vi "RunJS.vi"() -> ()   [LabVIEW 2013]
uses:
  E:/Dropbox/ni/lvcef/github/lvcef/dotnet/LVCef/bin/Debug/LVCef.dll
  dotnet/LVCef/bin/Debug/LVCef.dll
panel:
  in  "LVCefControl":refnum<k24>(container)
  out "Numeric":i32
  in  "stop":bool
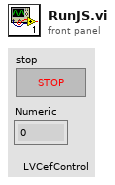
[diagram p1: front panel]
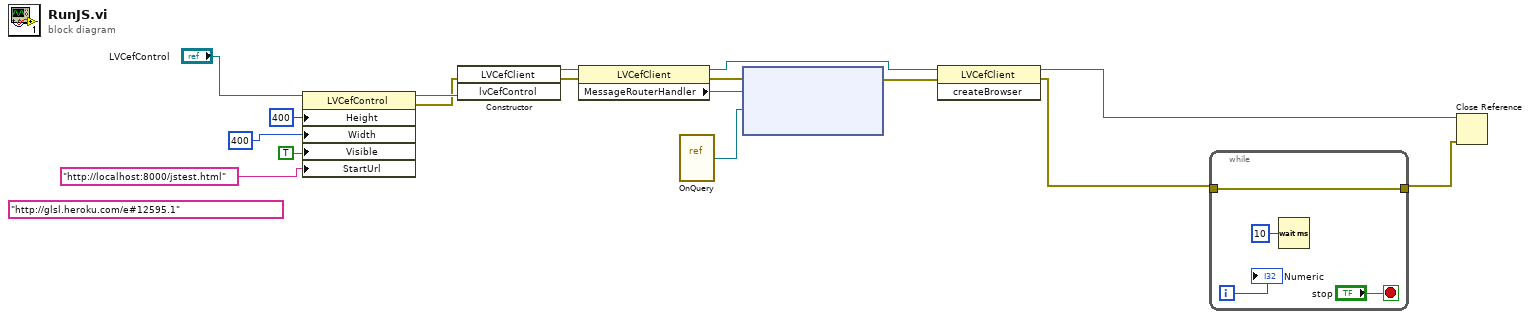
[diagram p0: block diagram]
diagram:
  (unwired) "http://glsl.heroku.com/e#12595.1" ("StartUrl")
  n1 = property class="LVCefControl"(reference="LVCefControl", "Height"=400, "Width"=400, "Visible"=TRUE, "StartUrl"="http://localhost:8000/jstest.html") -> (reference out=w13:refnum<k24>, error out=w12:errorcluster)  [unwired: 1 in]
  n2 = constructor class="LVCefClient"(error in=w12, "lvCefControl"=w13) -> (reference out=w7:refnum<k24>, error out=w8:errorcluster)  [unwired: 2 in, 2 out]
  n3 = property class="LVCefClient"(reference=w7, error in=w8) -> (reference out=w3:refnum<k24>, error out=w6:errorcluster, "MessageRouterHandler"=w5:refnum<k24>)
  n4 = vi-ref "OnQuery.vi"() -> (w1:refnum<vi>)
  n5 = node(w6, w5, w1) -> (w4:errorcluster)  [unwired: 2 in, 1 out]
  n6 = invoke class="LVCefClient" method="createBrowser"(reference=w3, error in=w4) -> (reference out=w9:refnum<k24>, error out=w11:errorcluster)  [unwired: 1 in, 1 out]
  n7 = while {
    tunnel: w11 -> [w18]
    tunnel: [w18] -> w10
    i -> [w20]
    stop <- "stop" stop-if-true
    n8 = Wait (ms)(milliseconds to wait=u32 10) -> ()  [unwired: 1 out]
    "Numeric" <- w20
  }
  n9 = Close Reference(reference=w9, error in (no error)=w10) -> ()  [unwired: 1 out]
